vi "Read Horizontal Offset.vi"(8 "error in (no error)":errorcluster, 10 "Channel Name":string, 11 "Scope in":refnum<class "Scope.lvclass">) -> (0 "error out":errorcluster, 1 "Offset (s)":dbl, 3 "Scope out":refnum<class "Scope.lvclass">)   [LabVIEW 2015, in "Scope.lvclass"]
uses:
  Scope.lvclass
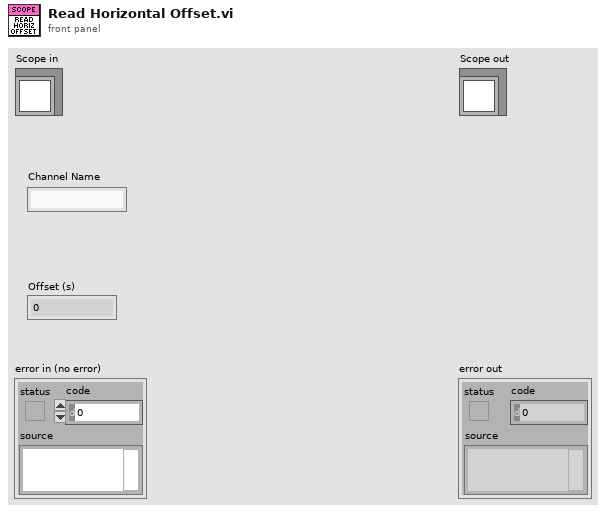
[diagram p1: front panel]
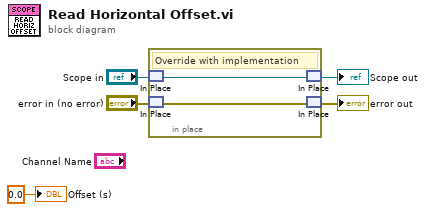
[diagram p0: block diagram]
diagram:
  n1 = in-place {
    # "Override with implementation"
    n2 = in-place-match #1("Scope in") -> (w7:refnum<class "Scope.lvclass">)
    n3 = in-place-match #2("error in (no error)") -> (w6:errorcluster)
    n4 = in-place-match #1(w7) -> (→"Scope out":refnum<class "Scope.lvclass">)
    n5 = in-place-match #2(w6) -> (→"error out":errorcluster)
  }
  "Offset (s)" <- 0.0 ("Offset (s)")
